vi "CLIENT.vi"() -> ()   [LabVIEW 2019]
panel:
  out "data out":string
  out "error out":errorcluster
  in  "stop":bool
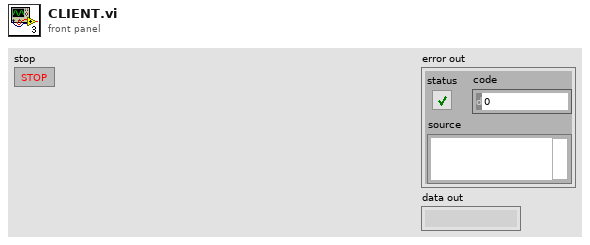
[diagram p1: front panel]
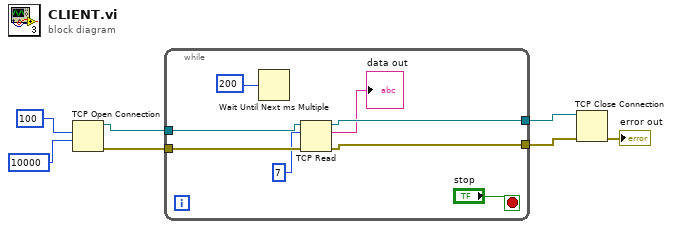
[diagram p0: block diagram]
diagram:
  n1 = TCP Open Connection(remote port or service name=u16 100, timeout ms (60000)=10000) -> (connection ID=w7:refnum<k5>, error out=w5:errorcluster)  [unwired: 3 in]
  n2 = while {
    tunnel: w7 -> [w14]
    tunnel: [w13] -> w6
    tunnel: w5 -> [w12]
    tunnel: [w11] -> w4
    stop <- "stop" stop-if-true
    n3 = Wait Until Next ms Multiple(millisecond multiple=u32 200 ("millisecond timer value")) -> ()  [unwired: 1 out]
    n4 = TCP Read(connection ID=w14, bytes to read=7, error in (no error)=w12) -> (connection ID out=w13:refnum<k5>, data out=→"data out":string, error out=w11:errorcluster)  [unwired: 2 in]
  }
  n5 = TCP Close Connection(connection ID=w6, error in (no error)=w4) -> (error out=→"error out":errorcluster)  [unwired: 1 in, 1 out]
